vi "Task Loop.vi"(8 "error in (no error)":errorcluster, 11 "VolatusCoreTask in":refnum<class "VolatusCoreTask.lvclass">) -> (0 "error out":errorcluster)   [LabVIEW 2020, in "Volatus.lvlib" / "VolatusCoreTask.lvclass"]
uses:
  VolatusCoreTask.lvclass
  VolatusCoreTask.lvclass/VolatusCoreTask.ctl
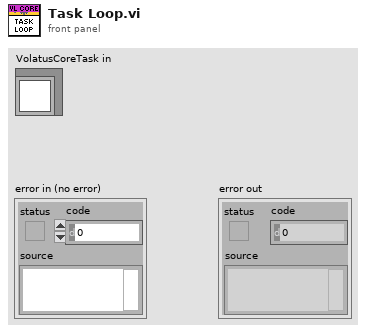
[diagram p1: front panel]
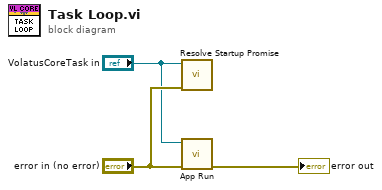
[diagram p0: block diagram]
diagram:
  n1 = call "Resolve Startup Promise.vi"("error in (no error)"="error in (no error)", "VolatusCoreTask in"="VolatusCoreTask in") -> ()  [unwired: 8 in, 2 out]
  n2 = call "App Run.vi"("error in (no error)"="error in (no error)", "VolatusCoreTask in"="VolatusCoreTask in") -> ("error out"=→"error out":errorcluster)  [unwired: 8 in, 1 out]
